vi "DAQmx Read (Digital Wfm 1Chan NSamp).vi"(0 "task/channels in":refnum<k21>, 7 "number of samples per channel":i32=-1, 9 "timeout":dbl=10.0 format="%0.2f", 11 "error in":errorcluster) -> (4 "task out":refnum<k21>, 6 "data":digitalwaveform(waveform)={"t0"=timestamp(0 s since 1904-01-01), "dt"=0.0, "Y"={"transitions"=[], "data"=[]}, "error"={"status"=FALSE, "code"=37421928, "source"=""}}, 15 "error out":errorcluster)   [LabVIEW 2011]
doc: "Reads a digital waveform from a task that contains a single digital input channel."
uses:
  nilvaiu.dll
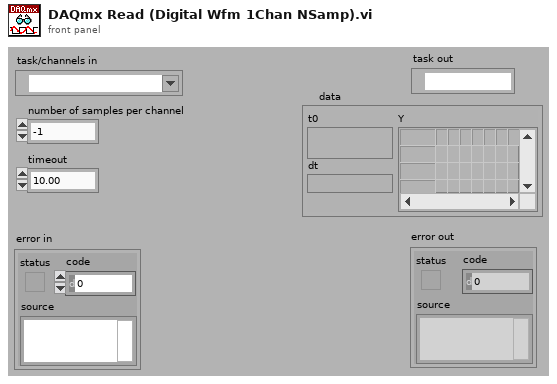
[diagram p1: front panel]
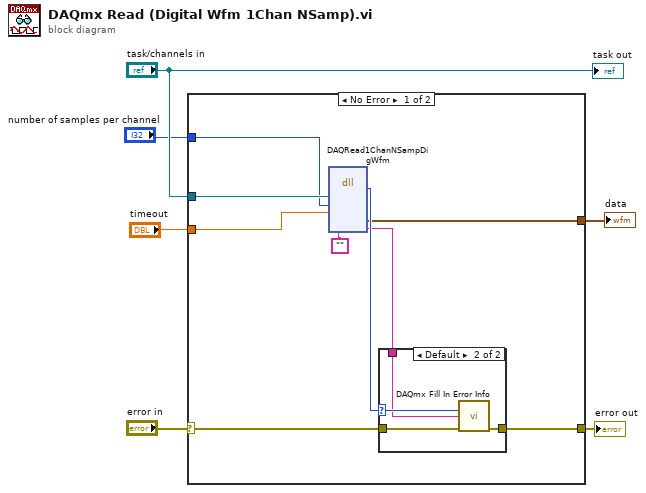
[diagram p0: block diagram]
diagram:
  n1 = case shown="No Error" "error in" {
    selector: "error in" -> [w9 w21]
    tunnel: [w13 w21] -> w5
    tunnel: "task/channels in" -> [w15 _]
    tunnel: [w10 _] -> w3
    tunnel: "number of samples per channel" -> [w8 _]
    tunnel: "timeout" -> [w7 _]
    frame No Error {
      n2 = dll-call lib="nilvaiu.*" fn="DAQRead1ChanNSampDigWfm"("taskID"=w15, "numberOfSamples"=w8, "timeout"=w7, "extendedErrorInfo"="") -> (w14:i32, "data"=w10:digitalwaveform, "extendedErrorInfo"=w11:string)  [unwired: 5 in, 4 out]
      n3 = case shown="Default" w14 {
        selector: w14 -> [_ w18]
        tunnel: w9 -> [w16 w20]
        tunnel: [w16 w19] -> w13
        tunnel: w11 -> [_ w17]
        frame 0 {
        }
        frame Default {
          n4 = call "DAQmx Fill In Error Info.vi"("status code"=w18, "extended error info"=w17, "error in"=w20) -> ("error out"=w19:errorcluster)  [unwired: 1 in, 11 out]
        }
      }
    }
    frame Error {
    }
  }
  "error out" <- w5
  "data" <- w3
  "task out" <- "task/channels in"
